vi "Dashboard Main.vi"() -> ()   [LabVIEW 2013]
uses:
  Program Files (x86)/National Instruments/LabVIEW 2013/examples/FRC/Vision/2014 Target Detection/TargetType.ctl
  <vilib>/event_ctls.llb/eventvkey.ctl
  <vilib>/Rock Robotics/WPI/Dashboard/WPI_DashboardLogging Global.vi
  <vilib>/Utility/config.llb/Write Key (String).vi
  <vilib>/Utility/config.llb/Write Key (I32).vi
  <vilib>/Utility/config.llb/NI_LVConfig.lvlib
panel:
  in  "Score Limit":dbl
  out "Target Info":T2(array[cluster])
  in  "Area Size Limit %":dbl=0.06 format="%#_13g"
  out "Image Message":string="Timeout in Camera Communications"
  in  "Rec Mode":enum32{"Stop", "Record", "Playback"}(radio)
  in  "Dashboard Tab":T3(tab)=enum."Auto"
  in  "Camera Settings":T4={"Frame Rate"=30, "Compression"=30, "Size"=1} {"Frame Rate" scale=1.0..30.0; "Size" items=["640x480", "320x240", "160x120"]}
  out "MotorSliders R":cluster{"MotorSlide1":dbl, "MotorSlide2":dbl} {"MotorSlide2" scale=-1.0..1.0 scale format="%#_2e"; "MotorSlide1" scale=-1.0..1.0 scale format="%#_2e"}
  out "MotorChart R":cluster{"Numeric":dbl, "Numeric":dbl}(graph)
  out "MotorSliders L":T5 {"MotorSlide4 2" scale=0.0..14.0 scale format="%#_2e"; "MotorSlide2" scale=-1.0..1.0 scale format="%#_2e"; "MotorSlide1" scale=-1.0..1.0 scale format="%#_2e"}
  out "MotorChart L":T6(graph)
  out "JS1 Z":dbl(slide) scale=-1.0..1.0 scale format="%#_2e"
  out "Joystick 1":cluster{"X":dbl, "Y":dbl}[](graph)
  out "JS Buttons 1":T7
  out "JS2 Z":dbl(slide) scale=-1.0..1.0 scale format="%#_2e"
  out "Joystick 2":cluster{"X":dbl, "Y":dbl}[](graph)
  out "JS Buttons 2":T7
  out "Mode":T8(ring)=enum."Auto Disabled"
  out "Camera IP":string
  in  "DB Camera Config":bool
  out "fps":dbl format="%#.1g"
  out "Mbps":dbl format="%#.1g"
  out "Mbps 2":bool
  out "LED 1":bool
  in  "Slider 1":dbl(slide) scale=0.0..100.0
  in  "Left?":bool
  in  "Checkbox 2":bool
  in  "Checkbox 1":bool
  in  "Color Components":T9={"Hue"={142.0, 183.0}, "Sat"={188.0, 255.0}, "Val"={0.0, 255.0}} {"Val" scale=0.0..255.0; "Sat" scale=0.0..255.0; "Hue" scale=0.0..255.0 scale format="%#_3g"}
  in  "Std Devs":cluster{"Hue":dbl, "Sat":dbl, "Val":dbl}={"Hue"=4.0, "Sat"=6.0, "Val"=4.0}
  in  "Score Cutoff":dbl(slide)=54.248366013071895 scale=0.0..100.0
  out "Distances":T10(array[cluster])
  out "State":T1
  in  "Test Slider":dbl(slide) scale=0.0..100.0 scale format="%#_3g"
  in  "On/Off":bool caption="Solenoid"
  in  "Test Name":u16(ring) items=["Select the test to run...", "Example Test", "-------------------------------", "List of tests is built in robot code.", "Replace with your own automated tests."]
  in  "Test Tree":string(tree)
  in  "Motor":cluster{"Value":dbl, "Enable":bool} {"Value" scale=-1.0..1.0 scale format="%#_3g"}
  out "Progress":T11 {"Test Progress" scale=0.0..100.0}
  in  "Rev/Fwd":cluster{"Forward":bool, "Reverse":bool}
  in  "Test Ring":u16(ring) items=["Auto", "Fixed indoor", "Fixed outdoor 1", "Fixed outdoor 2", "Fixed fluorescent 1", "Fixed fluorescent 2", "Hold current"]
  in  "Listbox":i32(listbox)
  out "Tree":string(tree)
  out "Camera Image":T12(plugin-control)
  in  "Enable":bool=TRUE
  # "Left"
  # "Front"
  # "Right"
  # "Battery"
  # "Customize by placing controls and indicators here and name to\nmatch Dashboard Variables on robot."
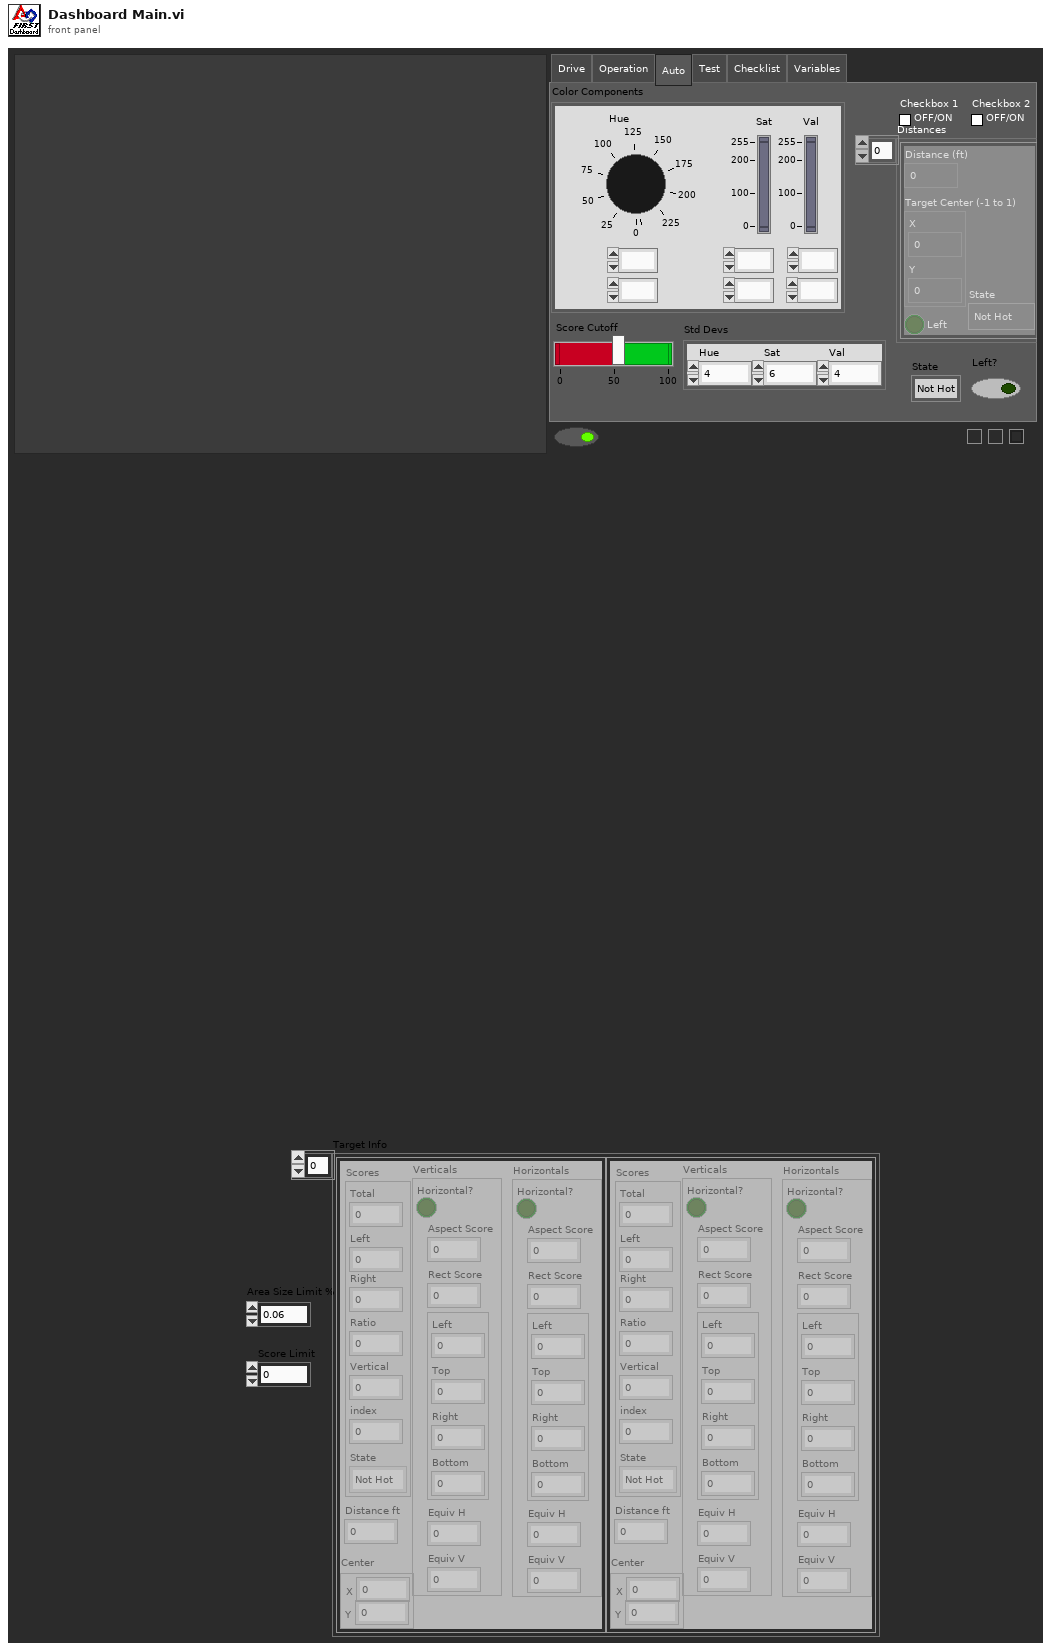
[diagram p1: front panel]
types:
  T1 = typedef "TargetType.ctl" = enum16{"Not Hot", "Hot"}
  T2 = cluster{"Scores":cluster{"Total":dbl, "Left":dbl, "Right":dbl, "Ratio":dbl, "Vertical":dbl, "index":i32, "State":T1}, "Verticals":cluster{"Horizontal?":bool, "Aspect Score":dbl, "Rect Score":dbl, cluster{"Left":dbl, "Top":dbl, "Right":dbl, "Bottom":dbl}, "Equiv H":dbl, "Equiv V":dbl}, "Horizontals":cluster{"Horizontal?":bool, "Aspect Score":dbl, "Rect Score":dbl, cluster{"Left":dbl, "Top":dbl, "Right":dbl, "Bottom":dbl}, "Equiv H":dbl, "Equiv V":dbl}, "Distance ft":dbl, "Center":cluster{"X":dbl, "Y":dbl}}[]
  T3 = enum32{"Drive", "Operation", "Auto", "Test", "Checklist", "Variables"}
  T4 = cluster{"Frame Rate":i32, "Compression":i32, "Size":u16}
  T5 = cluster{"MotorSlide1":dbl, "MotorSlide2":dbl, "MotorSlide4 2":dbl}
  T6 = cluster{"Numeric":dbl, "Numeric":dbl, "Battery":sgl}
  T7 = cluster{bool, bool, bool, bool, bool, bool, bool, bool, bool, bool, bool, bool}
  T8 = enum8{"Tele-Op Disabled", "Tele-Op Enabled", "Auto Disabled", "Auto Enabled", "Test Disabled", "Test Enabled", ""}
  T9 = cluster{"Hue":cluster{dbl, dbl}, "Sat":cluster{dbl, dbl}, "Val":cluster{dbl, dbl}}
  T10 = cluster{"Distance (ft)":dbl, "Target Center (-1 to 1)":cluster{"X":dbl, "Y":dbl}, "Left":bool, "State":T1}[]
  T11 = cluster{"Test Progress":u8, "Test Progress Text":string}
  T12 = typedef "IMAQ Image.ctl" = refnum<image>
  T13 = typedef "Image Type" = u32
  T14 = cluster{"Horizontal":bool, "Aspect Score":dbl, "Rect Score":dbl, cluster{"Left":dbl, "Top":dbl, "Right":dbl, "Bottom":dbl}, "Equiv H":dbl, "Equiv V":dbl}[]
  T15 = cluster{"Scores":cluster{"Total":dbl, "Left":dbl, "Right":dbl, "Ratio":dbl, "Vertical":dbl, "index":i32, "State":T1}, "Verticals":cluster{"Horizontal?":bool, "Aspect Score":dbl, "Rect Score":dbl, cluster{"Left":dbl, "Top":dbl, "Right":dbl, "Bottom":dbl}, "Equiv H":dbl, "Equiv V":dbl}, "Horizontals":cluster{"Horizontal?":bool, "Aspect Score":dbl, "Rect Score":dbl, cluster{"Left":dbl, "Top":dbl, "Right":dbl, "Bottom":dbl}, "Equiv H":dbl, "Equiv V":dbl}, "Validated":bool}[]
  T16 = cluster{"Scores":cluster{"Total":dbl, "Left":dbl, "Right":dbl, "Ratio":dbl, "Vertical":dbl, "index":i32, "State":T1}, "Verticals":cluster{"Horizontal?":bool, "Aspect Score":dbl, "Rect Score":dbl, cluster{"Left":dbl, "Top":dbl, "Right":dbl, "Bottom":dbl}, "Equiv H":dbl, "Equiv V":dbl}, "Horizontals":cluster{"Horizontal?":bool, "Aspect Score":dbl, "Rect Score":dbl, cluster{"Left":dbl, "Top":dbl, "Right":dbl, "Bottom":dbl}, "Equiv H":dbl, "Equiv V":dbl}, "Distance (ft)":dbl, "Target Center (-1 to 1)":cluster{"X":dbl, "Y":dbl}}[]
  T17 = cluster{"Target Info[0]":cluster{"Scores":cluster{"Total":dbl, "Left":dbl, "Right":dbl, "Ratio":dbl, "Vertical":dbl, "index":i32, "State":T1}, "Verticals":cluster{"Horizontal?":bool, "Aspect Score":dbl, "Rect Score":dbl, cluster{"Left":dbl, "Top":dbl, "Right":dbl, "Bottom":dbl}, "Equiv H":dbl, "Equiv V":dbl}, "Horizontals":cluster{"Horizontal?":bool, "Aspect Score":dbl, "Rect Score":dbl, cluster{"Left":dbl, "Top":dbl, "Right":dbl, "Bottom":dbl}, "Equiv H":dbl, "Equiv V":dbl}, "Distance (ft)":dbl, "Target Center (-1 to 1)":cluster{"X":dbl, "Y":dbl}}, "Target Info[1]":cluster{"Scores":cluster{"Total":dbl, "Left":dbl, "Right":dbl, "Ratio":dbl, "Vertical":dbl, "index":i32, "State":T1}, "Verticals":cluster{"Horizontal?":bool, "Aspect Score":dbl, "Rect Score":dbl, cluster{"Left":dbl, "Top":dbl, "Right":dbl, "Bottom":dbl}, "Equiv H":dbl, "Equiv V":dbl}, "Horizontals":cluster{"Horizontal?":bool, "Aspect Score":dbl, "Rect Score":dbl, cluster{"Left":dbl, "Top":dbl, "Right":dbl, "Bottom":dbl}, "Equiv H":dbl, "Equiv V":dbl}, "Distance (ft)":dbl, "Target Center (-1 to 1)":cluster{"X":dbl, "Y":dbl}}, "Target Info[2]":cluster{"Scores":cluster{"Total":dbl, "Left":dbl, "Right":dbl, "Ratio":dbl, "Vertical":dbl, "index":i32, "State":T1}, "Verticals":cluster{"Horizontal?":bool, "Aspect Score":dbl, "Rect Score":dbl, cluster{"Left":dbl, "Top":dbl, "Right":dbl, "Bottom":dbl}, "Equiv H":dbl, "Equiv V":dbl}, "Horizontals":cluster{"Horizontal?":bool, "Aspect Score":dbl, "Rect Score":dbl, cluster{"Left":dbl, "Top":dbl, "Right":dbl, "Bottom":dbl}, "Equiv H":dbl, "Equiv V":dbl}, "Distance (ft)":dbl, "Target Center (-1 to 1)":cluster{"X":dbl, "Y":dbl}}, "Target Info[3]":cluster{"Scores":cluster{"Total":dbl, "Left":dbl, "Right":dbl, "Ratio":dbl, "Vertical":dbl, "index":i32, "State":T1}, "Verticals":cluster{"Horizontal?":bool, "Aspect Score":dbl, "Rect Score":dbl, cluster{"Left":dbl, "Top":dbl, "Right":dbl, "Bottom":dbl}, "Equiv H":dbl, "Equiv V":dbl}, "Horizontals":cluster{"Horizontal?":bool, "Aspect Score":dbl, "Rect Score":dbl, cluster{"Left":dbl, "Top":dbl, "Right":dbl, "Bottom":dbl}, "Equiv H":dbl, "Equiv V":dbl}, "Distance (ft)":dbl, "Target Center (-1 to 1)":cluster{"X":dbl, "Y":dbl}}, "Target Info[4]":cluster{"Scores":cluster{"Total":dbl, "Left":dbl, "Right":dbl, "Ratio":dbl, "Vertical":dbl, "index":i32, "State":T1}, "Verticals":cluster{"Horizontal?":bool, "Aspect Score":dbl, "Rect Score":dbl, cluster{"Left":dbl, "Top":dbl, "Right":dbl, "Bottom":dbl}, "Equiv H":dbl, "Equiv V":dbl}, "Horizontals":cluster{"Horizontal?":bool, "Aspect Score":dbl, "Rect Score":dbl, cluster{"Left":dbl, "Top":dbl, "Right":dbl, "Bottom":dbl}, "Equiv H":dbl, "Equiv V":dbl}, "Distance (ft)":dbl, "Target Center (-1 to 1)":cluster{"X":dbl, "Y":dbl}}, "Target Info[5]":cluster{"Scores":cluster{"Total":dbl, "Left":dbl, "Right":dbl, "Ratio":dbl, "Vertical":dbl, "index":i32, "State":T1}, "Verticals":cluster{"Horizontal?":bool, "Aspect Score":dbl, "Rect Score":dbl, cluster{"Left":dbl, "Top":dbl, "Right":dbl, "Bottom":dbl}, "Equiv H":dbl, "Equiv V":dbl}, "Horizontals":cluster{"Horizontal?":bool, "Aspect Score":dbl, "Rect Score":dbl, cluster{"Left":dbl, "Top":dbl, "Right":dbl, "Bottom":dbl}, "Equiv H":dbl, "Equiv V":dbl}, "Distance (ft)":dbl, "Target Center (-1 to 1)":cluster{"X":dbl, "Y":dbl}}, "Target Info[6]":cluster{"Scores":cluster{"Total":dbl, "Left":dbl, "Right":dbl, "Ratio":dbl, "Vertical":dbl, "index":i32, "State":T1}, "Verticals":cluster{"Horizontal?":bool, "Aspect Score":dbl, "Rect Score":dbl, cluster{"Left":dbl, "Top":dbl, "Right":dbl, "Bottom":dbl}, "Equiv H":dbl, "Equiv V":dbl}, "Horizontals":cluster{"Horizontal?":bool, "Aspect Score":dbl, "Rect Score":dbl, cluster{"Left":dbl, "Top":dbl, "Right":dbl, "Bottom":dbl}, "Equiv H":dbl, "Equiv V":dbl}, "Distance (ft)":dbl, "Target Center (-1 to 1)":cluster{"X":dbl, "Y":dbl}}, "Target Info[7]":cluster{"Scores":cluster{"Total":dbl, "Left":dbl, "Right":dbl, "Ratio":dbl, "Vertical":dbl, "index":i32, "State":T1}, "Verticals":cluster{"Horizontal?":bool, "Aspect Score":dbl, "Rect Score":dbl, cluster{"Left":dbl, "Top":dbl, "Right":dbl, "Bottom":dbl}, "Equiv H":dbl, "Equiv V":dbl}, "Horizontals":cluster{"Horizontal?":bool, "Aspect Score":dbl, "Rect Score":dbl, cluster{"Left":dbl, "Top":dbl, "Right":dbl, "Bottom":dbl}, "Equiv H":dbl, "Equiv V":dbl}, "Distance (ft)":dbl, "Target Center (-1 to 1)":cluster{"X":dbl, "Y":dbl}}, "Target Info[8]":cluster{"Scores":cluster{"Total":dbl, "Left":dbl, "Right":dbl, "Ratio":dbl, "Vertical":dbl, "index":i32, "State":T1}, "Verticals":cluster{"Horizontal?":bool, "Aspect Score":dbl, "Rect Score":dbl, cluster{"Left":dbl, "Top":dbl, "Right":dbl, "Bottom":dbl}, "Equiv H":dbl, "Equiv V":dbl}, "Horizontals":cluster{"Horizontal?":bool, "Aspect Score":dbl, "Rect Score":dbl, cluster{"Left":dbl, "Top":dbl, "Right":dbl, "Bottom":dbl}, "Equiv H":dbl, "Equiv V":dbl}, "Distance (ft)":dbl, "Target Center (-1 to 1)":cluster{"X":dbl, "Y":dbl}}}
  T18 = cluster{cluster{dbl, dbl}, cluster{dbl, dbl}, cluster{dbl, dbl}}
  T19 = cluster{"Scores":cluster{"Total":dbl, "Left":dbl, "Right":dbl, "Ratio":dbl, "Vertical":dbl, "index":i32, "State":T1}, "Verticals":cluster{"Horizontal?":bool, "Aspect Score":dbl, "Rect Score":dbl, cluster{"Left":dbl, "Top":dbl, "Right":dbl, "Bottom":dbl}, "Equiv H":dbl, "Equiv V":dbl}, "Horizontals":cluster{"Horizontal?":bool, "Aspect Score":dbl, "Rect Score":dbl, cluster{"Left":dbl, "Top":dbl, "Right":dbl, "Bottom":dbl}, "Equiv H":dbl, "Equiv V":dbl}, "Distance (ft)":dbl, "Target Center (-1 to 1)":cluster{"X":dbl, "Y":dbl}}
  T20 = cluster{"Total":dbl, "Left":dbl, "Right":dbl, "Ratio":dbl, "Vertical":dbl, "index":i32, "State":T1}
  T21 = cluster{"Digital Inputs":bool[], "Digital Outputs":bool[]}
  T22 = cluster{"Competition mode":bool, "Robot Link":bool, "Autonomous":bool, "Enabled":bool, "E-Stop":bool, "Simulated":bool, "TestMode":bool, "Docked Window":bool}
  T23 = cluster{"Boolean Array[0]":bool, "Boolean Array[1]":bool, "Boolean Array[2]":bool, "Boolean Array[3]":bool, "Boolean Array[4]":bool, "Boolean Array[5]":bool, "Boolean Array[6]":bool, "Boolean Array[7]":bool, "Boolean Array[8]":bool, "Boolean Array[9]":bool, "Boolean Array[10]":bool, "Boolean Array[11]":bool}
  T24 = typedef "NI_LVConfig.lvlib/Config Data RefNum.ctl" = refnum<k1>
  T25 = typedef "eventvkey.ctl" = enum16{"ASCII", "Enter", "Return", "Shift", "Ctrl", "Alt", "Cmd", "Opt", "Caps", "NumLock", "Clear", "Break", "Up", "Down", "Left", "Right", "Insert", "Delete", "Home", "End", "PageUp", "PageDown", "Escape", "Help", "Pause", "ScrollLock", "F1", "F2", "F3", "F4", "F5", "F6", "F7", "F8", "F9", "F10", "F11", "F12", "F13", "F14", "F15", "F16", "F17", "F18", "F19", "F20", "F21", "F22", "F23", "F24", "Play", "VolumeUp", "VolumeDown", "Mute", "Two Byte Char"}
  T26 = cluster{"Image Size":bool, "Image Type":bool, "Pixel Value":bool, "ROI Information":bool, "Zoom Factor":bool}
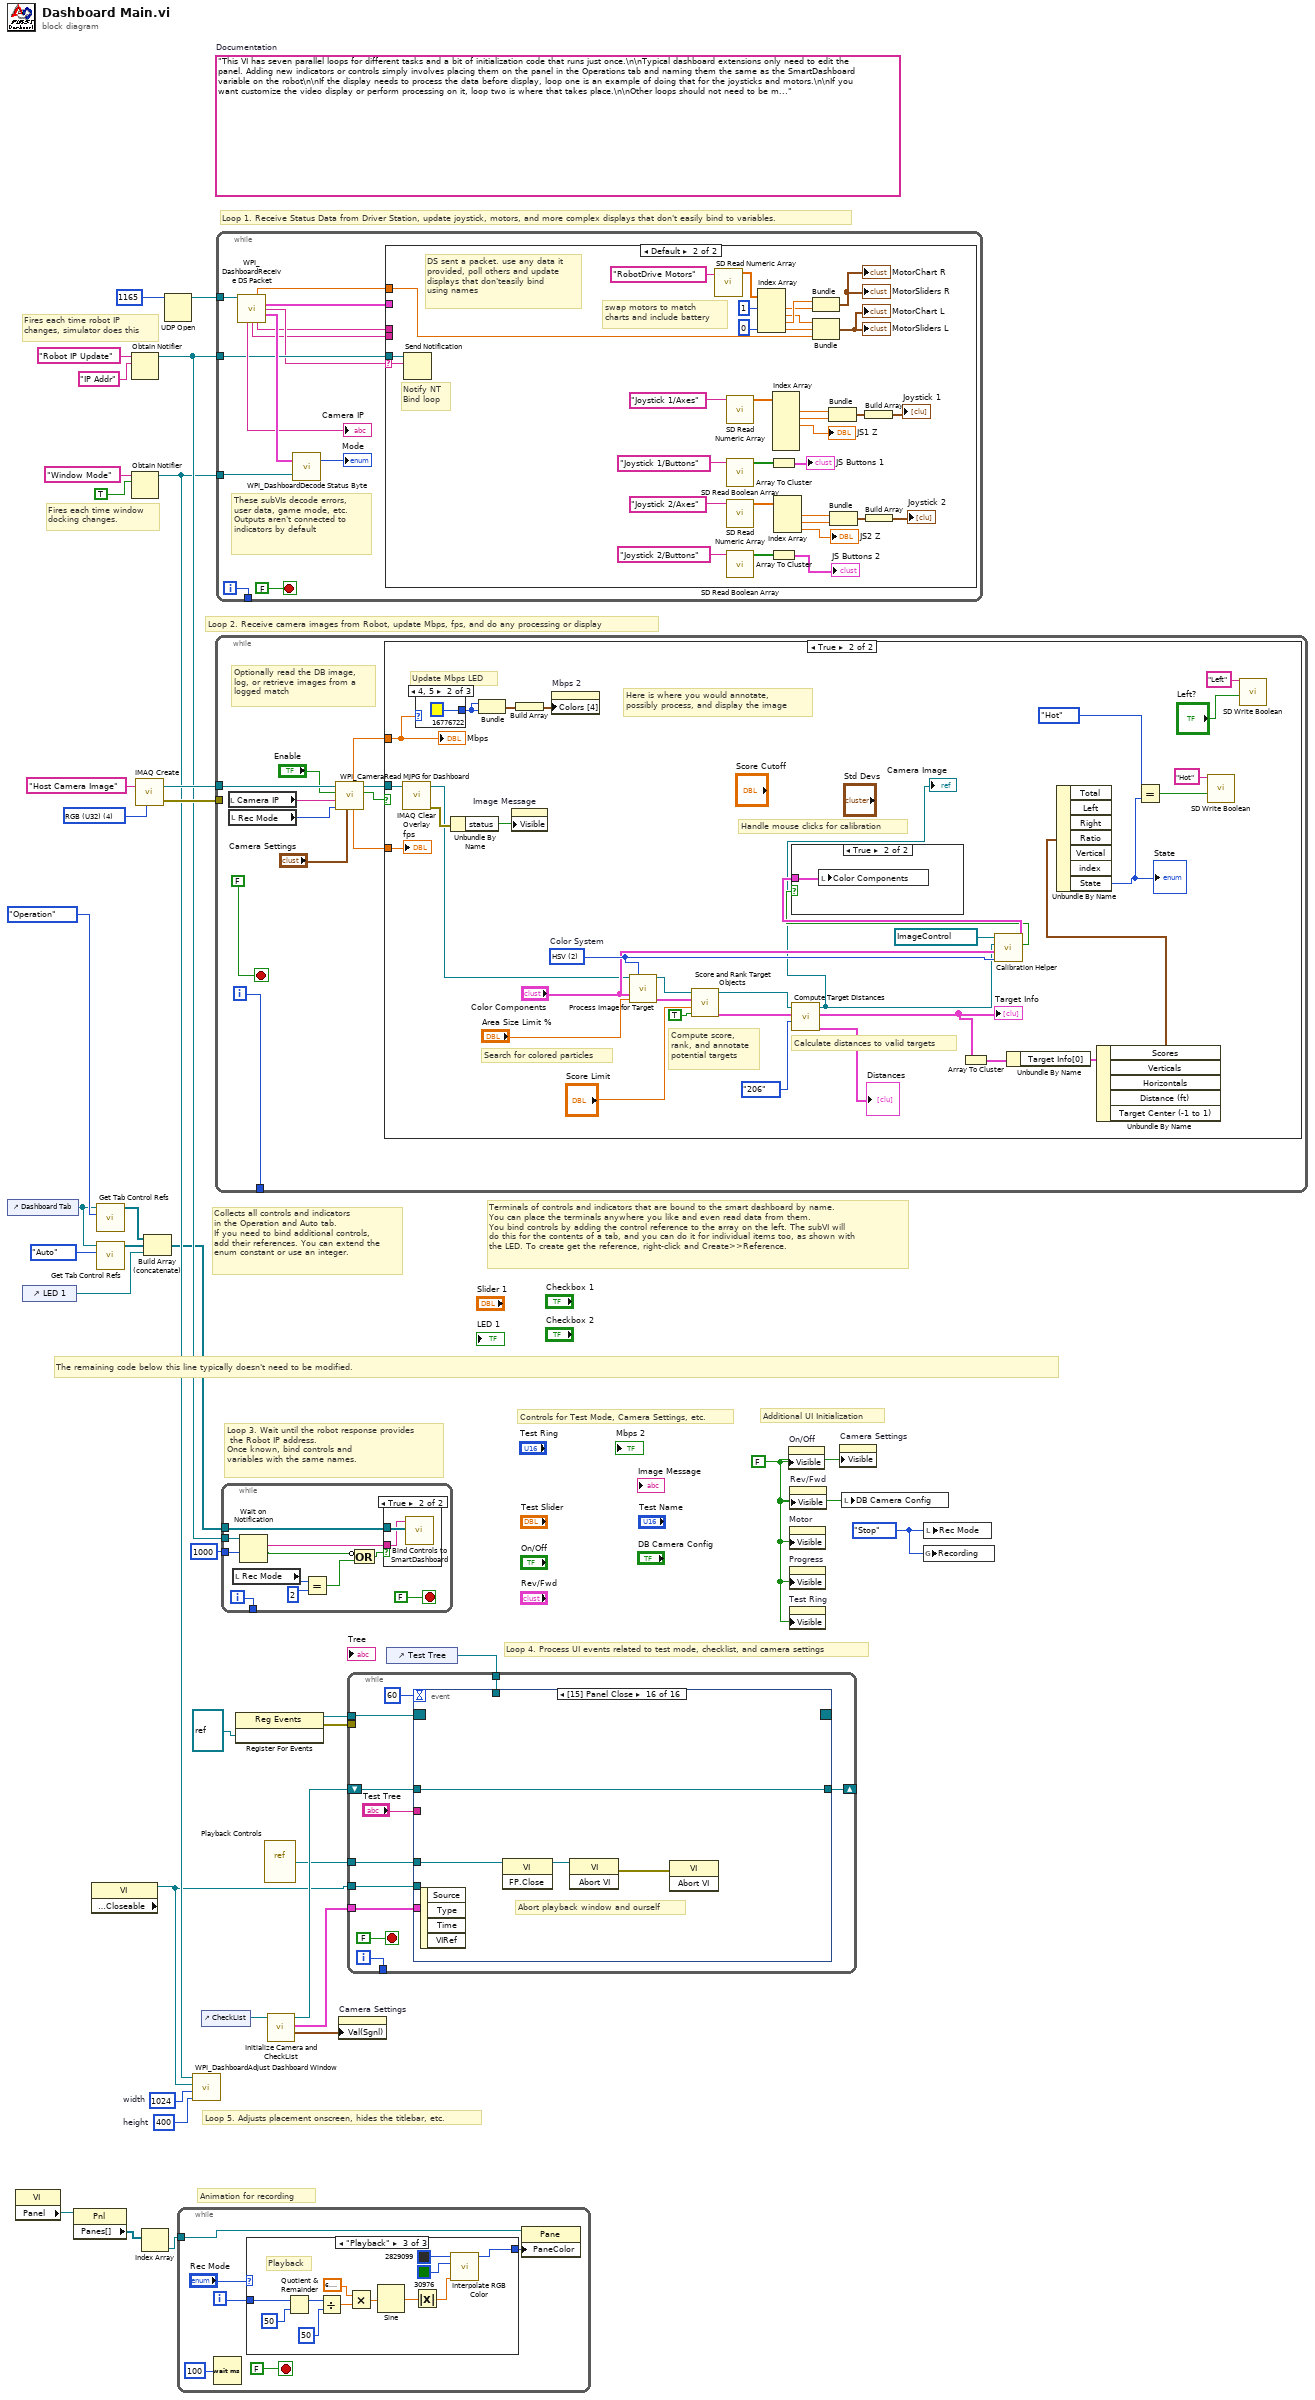
[diagram p0: block diagram]
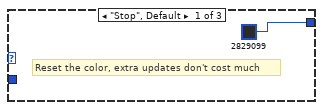
[diagram p2: hidden frame]
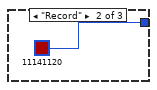
[diagram p3: hidden frame]
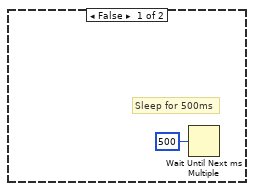
[diagram p5: hidden frame]
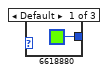
[diagram p7: hidden frame]
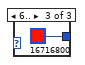
[diagram p8: hidden frame]
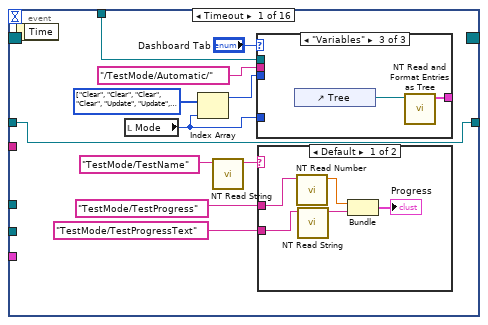
[diagram p9: hidden frame]
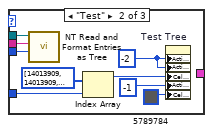
[diagram p11: hidden frame]
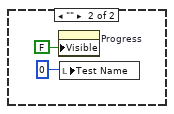
[diagram p12: hidden frame]
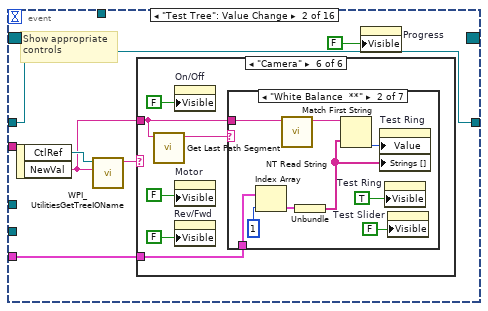
[diagram p13: hidden frame]
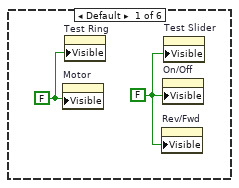
[diagram p14: hidden frame]
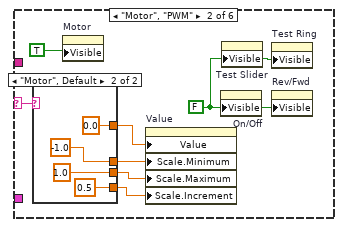
[diagram p15: hidden frame]
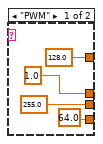
[diagram p16: hidden frame]
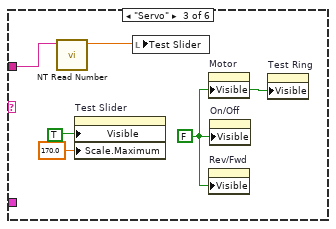
[diagram p17: hidden frame]
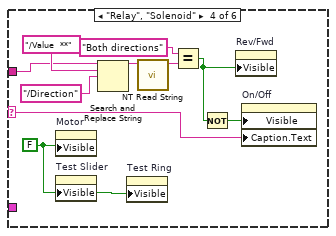
[diagram p18: hidden frame]
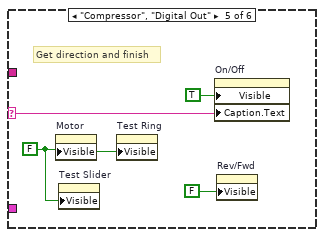
[diagram p19: hidden frame]
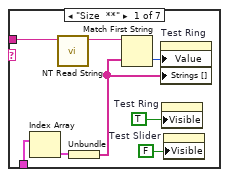
[diagram p20: hidden frame]
diagram:
  w8 = enum32{"Stop", "Record", "Playback"}."Stop" ("Rec Mode")
  w11 = 400  # height
  w12 = 1024  # width
  w25 = FALSE ("Visible")
  (unwired) "This VI has seven parallel loops for different tasks and a bit of initialization code that runs just once.\n\nTypical dashboard extensions only need to edit the panel. Adding new indicators or controls simply involves placing them on the panel in the Operations tab and naming them the same as the SmartDashboard variable on the robot\n\nIf the display needs to process the data before display, loop one is an example of doing that for the joysticks and motors.\n\nIf you want customize the video display or perform processing on it, loop two is where that takes place.\n\nOther loops should not need to be modified. They are pretty standard, and document the task they perform."  # Documentation
  w35 = T13 4 items=["Grayscale (U8)", "Grayscale (I16)", "Grayscale (SGL)", "Complex (CSG)", "RGB (U32)", "HSL (U32)", "RGB (U64)"] ("Image Type")
  # "Controls for Test Mode, Camera Settings, etc."
  # "Additional UI Initialization"
  # "Animation for recording"
  # "Fires each time robot IP\nchanges, simulator does this"
  # "Fires each time window\ndocking changes."
  # "Collects all controls and indicators\nin the Operation and Auto tab.\nIf you need to bind additional controls,\nadd their references. You can extend the\nenum constant or use an integer."
  # "The remaining code below this line typically doesn't need to be modified."
  # "Loop 4. Process UI events related to test mode, checklist, and camera settings"
  # "Terminals of controls and indicators that are bound to the smart dashboard by name.\nYou can place the terminals anywhere you like and even read data from them.\nYou bind controls by adding the control reference to the array on the left. The subVI will\ndo this for the contents of a tab, and you can do it for individual items too, as shown with\nthe LED. To create get the reference, right-click and Create>>Reference."
  # "Loop 3. Wait until the robot response provides\n the Robot IP address.\nOnce known, bind controls and\nvariables with the same names."
  # "Loop 5. Adjusts placement onscreen, hides the titlebar, etc."
  # "Loop 1. Receive Status Data from Driver Station, update joystick, motors, and more complex displays that don't easily bind to variables."
  # "Loop 2. Receive camera images from Robot, update Mbps, fps, and do any processing or display"
  n1 = control-ref of="Dashboard Tab"() -> (w6:refnum<vi>)
  n2 = property class="VI"() -> ("Panel"=w19:refnum<vi>)  [unwired: 2 in, 2 out]
  n3 = control-ref of="LED 1"() -> (w1:refnum<vi>)
  n4 = property class="Pnl"(reference=w19) -> ("Panes[]"=w20:refnum<vi>[])  [unwired: 1 in, 2 out]
  n5 = property class="VI" props=["Front Panel.Closeable"]() -> (reference out=w7:refnum<vi>)  [unwired: 2 in, 2 out]
  n6 = call <vilib>:"Get Tab Control Refs.vi"("Page Index"=T3."Operation" ("Dashboard Tab"), "TabControl in"=w6) -> ("ControlsOnPage"=w4:refnum<vi>[])  [unwired: 9 in]
  n7 = call <vilib>:"Get Tab Control Refs.vi"("Page Index"=T3."Auto" ("Dashboard Tab"), "TabControl in"=w6) -> ("ControlsOnPage"=w5:refnum<vi>[])  [unwired: 9 in]
  n8 = Obtain Notifier(name (unnamed)="Robot IP Update", notification data type="IP Addr" ("name (unnamed)")) -> (notifier out=w29:refnum<notifier>)  [unwired: 2 in, 2 out]
  n9 = Obtain Notifier(name (unnamed)="Window Mode", notification data type=TRUE) -> (notifier out=w10:refnum<notifier>)  [unwired: 2 in, 2 out]
  n10 = call "IMAQ Create"("Image Name"="Host Camera Image", "Image Type"=w35) -> ("New Image"=w33:T12, "error out"=w32:errorcluster)  [unwired: 2 in, 1 out]
  n11 = Index Array(array=w20) -> (element=w18:refnum<vi>)  [unwired: 1 in]
  n12 = Build Array (concatenate)(w4, w5, w1) -> (w3:refnum<vi>[])
  n13 = UDP Open(11:u16 1165 ("port")) -> (port=w36:refnum<k16>)  [unwired: 2 in, 4 out]
  n14 = while {
    tunnel: w18 -> [w39]
    i -> [w42]
    stop <- FALSE stop-if-true
    n15 = Wait (ms)(milliseconds to wait=u32 100) -> ()  [unwired: 1 out]
    n16 = case shown="\"Playback\"" "Rec Mode" {
      tunnel: w42 -> [_ _ w57]
      tunnel: [u32 2829099 ("Base Color") u32 11141120 ("Target Color") w46] -> w38
      frame "Stop", Default {
        # "Reset the color, extra updates don't cost much"
      }
      frame "Record" {
      }
      frame "Playback" {
        # "Playback"
        n17 = Quotient & Remainder(x=w57, y=u32 50 ("milliseconds to wait")) -> (x-y*floor(x/y)=w53:u32)  [unwired: 1 out]
        n18 = Divide(x=w53, y=u32 50 ("milliseconds to wait")) -> (x/y=w50:dbl)
        n19 = Multiply(x=6.283185307179586, y=w50) -> (x*y=w55:dbl)
        n20 = Sine(x=w55) -> (sin(x)=w54:dbl)
        n21 = Absolute Value(x=w54) -> (abs(x)=w47:dbl)
        n22 = call "Interpolate RGB Color.vi"("Proportion"=w47, "Target Color"=u32 30976, "Base Color"=u32 2829099) -> ("Result Color"=w46:u32)  [unwired: 8 in]
      }
    }
    n23 = property class="Pane"(reference=w39, "PaneColor"=w38) -> ()  [unwired: 1 in, 2 out]
  }
  n24 = call <vilib>:"WPI_DashboardAdjust Dashboard Window.vi"("height"=w11, "width"=w12, "reference in"=w7, "Notifier in"=w10) -> ()  [unwired: 8 in]
  n25 = control-ref of="CheckList"() -> (w9:refnum<vi>)
  n26 = while {
    tunnel: w33 -> [w66]
    tunnel: w32 -> [_]
    tunnel: [w67] -> _
    i -> [w67]
    stop <- FALSE stop-if-true
    # "Optionally read the DB image,\nlog, or retrieve images from a\nlogged match"
    n27 = local read "Camera IP"() -> (w59:string)
    n28 = local read "Rec Mode"() -> (w58:enum32{"Stop", "Record", "Playback"})
    n29 = call <vilib>:"WPI_CameraRead MJPG for Dashboard.vi"("Camera Settings"="Camera Settings", "Rec Mode"=w58, "Camera IP"=w59, "Enable"="Enable", "Refnum in"=w66) -> ("Active"=w63:bool, "Refnum out"=w65:T12, "FPS"=w62:dbl, "Bandwidth (Mbps)"=w61:dbl)  [unwired: 3 in]
    n30 = case shown="True" w63 {
      tunnel: w65 -> [_ w98]
      tunnel: w61 -> [_ w97]
      tunnel: w62 -> [_ w96]
      frame False {
        # "Sleep for 500ms"
        n31 = Wait Until Next ms Multiple(millisecond multiple=u32 500) -> ()  [unwired: 1 out]
      }
      frame True {
        w91 = u16 2 items=["RGB", "HSL", "HSV", "HSI"]  # Color System
        # "Calculate distances to valid targets"
        # "Search for colored particles"
        # "Handle mouse clicks for calibration"
        # "Compute score,\nrank, and annotate\npotential targets"
        # "Here is where you would annotate,\npossibly process, and display the image"
        # "Update Mbps LED"
        n32 = call "IMAQ Clear Overlay"("Image"=w98) -> ("error out"=w102:errorcluster, "Image Out"=w86:T12)  [unwired: 2 in, 7 out]
        n33 = case shown="4, 5" w97 {
          tunnel: [u32 6618880 ("Color Box") u32 16776722 ("Color Box") u32 16716800 ("Color Box")] -> w99
          frame Default {
          }
          frame 4, 5 {
          }
          frame 6.. {
          }
        }
        n34 = Unbundle By Name(w102) -> ("status"=w103:bool)
        n35 = Bundle("Color Box"=w99, "Color Box"=w99) -> (w101:cluster{"Color Box":u32, "Color Box":u32})  [unwired: 1 out]
        n36 = property on="Image Message" class="Str"("Visible"=w103) -> ()  [unwired: 2 in, 2 out]
        n37 = Build Array(w101) -> (w100:cluster{"Color Box":u32, "Color Box":u32}[])
        n38 = property on="Mbps 2" class="Bool (strict)"("Colors [4]"=w100) -> ()  [unwired: 2 in, 2 out]
        n39 = call "Process Image for Target.vi"("Src Image"=w86, "Color Mode"=w91, "Color Components"="Color Components", "Area Cutoff %"="Area Size Limit %") -> ("Src Image Out"=w94:T12, "Particles"=w93:T14)  [unwired: 9 in, 1 out]
        n40 = call "Score and Rank Target Objects.vi"("Annotate"=TRUE, "Score Limit"="Score Limit", "Particles"=w93, "Image in"=w94) -> ("Target Info"=w92:T15, "Annotated Image"=w85:T12)  [unwired: 6 in]
        n41 = call "Compute Target Distances.vi"("Camera Type"=enum16{"206", "1011", "1013"}."206", "Target Info"=w92, "Image in"=w85) -> ("Distances"=→"Distances":T10, "Target Info"=w79:T16, "Image out"=w84:T12)  [unwired: 6 in]
        "Camera Image" <- w84
        "Target Info" <- w79
        n42 = Array To Cluster(array=w79) -> (cluster=w80:T17)
        n43 = call "Calibration Helper.vi"("Color Mode"=w91, "Color Components"="Color Components", "Image"=w84, "Image Ctl Refnum"=refnum<vi> refnum) -> ("Changed"=w88:bool, "output color"=w90:T18)  [unwired: 6 in]
        n44 = case shown="True" w88 {
          tunnel: w90 -> [_ w104]
          frame False {
          }
          frame True {
            n45 = local write "Color Components"(w104) -> ()
          }
        }
        n46 = Unbundle By Name(w80) -> ("Target Info[0]"=w78:T19)
        n47 = Unbundle By Name(w78) -> ("Scores"=w77:T20)  [unwired: 4 out]
        n48 = Unbundle By Name(w77) -> ("State"=w75:T1)  [unwired: 6 out]
        "State" <- w75
        n49 = Equal?(x=TargetType."Hot" ("State"), y=w75) -> (x = y?=w73:bool)
        n50 = call <vilib>:"SD Write Boolean.vi"("Boolean"=w73, "Name"="Hot") -> ()  [unwired: 8 in, 2 out]
        n51 = call <vilib>:"SD Write Boolean.vi"("Boolean"="Left?", "Name"="Left") -> ()  [unwired: 8 in, 2 out]
        "Mbps" <- w97
        "fps" <- w96
      }
    }
  }
  n52 = while {
    tunnel: w36 -> [w118]
    tunnel: w29 -> [w113]
    tunnel: w10 -> [w117]
    tunnel: [w114] -> _
    i -> [w114]
    stop <- FALSE stop-if-true
    # "These subVIs decode errors, user data, game mode, etc.\nOutputs aren't connected to indicators by default"
    n53 = call <vilib>:"WPI_DashboardReceive DS Packet.vi"("Recv Socket"=w118) -> ("Battery"=w108:sgl, "Driver Station"=w109:T21, "Robot IP Address"=w112:string, "Status"=w119:T22, "Camera IP Address"=→"Camera IP":string, "Low Priority User Data"=w111:string, "High Priority User Data"=w110:string)  [unwired: 1 in, 7 out]
    n54 = call <vilib>:"WPI_DashboardDecode Status Byte.vi"("Window Mode Notifier"=w117, "Status"=w119) -> ("Mode"=→"Mode":T8)  [unwired: 1 out]
    n55 = case shown="Default" w112 {
      selector: w112 -> [_ w131]
      tunnel: w113 -> [_ w132]
      tunnel: w111 -> [_ _]
      tunnel: w110 -> [_ _]
      tunnel: w109 -> [_ _]
      tunnel: w108 -> [_ w130]
      frame "0.0.0.0" {
        # "DS not sending packets, or no robot exists yet.\nDon't poll the variables"
      }
      frame Default {
        # "Notify NT\nBind loop"
        # "DS sent a packet. use any data it\nprovided, poll others and update\ndisplays that don'teasily bind\nusing names"
        # "swap motors to match\ncharts and include battery"
        n56 = Send Notification(notification=w131, notifier=w132) -> ()  [unwired: 1 in, 2 out]
        n57 = call <vilib>:"SD Read Numeric Array.vi"("Name"="RobotDrive Motors") -> ("Numeric Array"=w129:dbl[])  [unwired: 8 in, 2 out]
        n58 = call <vilib>:"SD Read Numeric Array.vi"("Name"="Joystick 1/Axes") -> ("Numeric Array"=w148:dbl[])  [unwired: 8 in, 2 out]
        n59 = call <vilib>:"SD Read Boolean Array.vi"("Name"="Joystick 1/Buttons") -> ("Boolean Array"=w150:bool[])  [unwired: 8 in, 2 out]
        n60 = call <vilib>:"SD Read Numeric Array.vi"("Name"="Joystick 2/Axes") -> ("Numeric Array"=w142:dbl[])  [unwired: 8 in, 2 out]
        n61 = call <vilib>:"SD Read Boolean Array.vi"("Name"="Joystick 2/Buttons") -> ("Boolean Array"=w141:bool[])  [unwired: 8 in, 2 out]
        n62 = Index Array(array=w129, index #1=1, index #4=0) -> (element #1=w125:dbl, element #2=w124:dbl, element #3=w126:dbl, element #4=w121:dbl)  [unwired: 2 in]
        n63 = Array To Cluster(array=w150) -> (cluster=→"JS Buttons 1":T23)
        n64 = Array To Cluster(array=w141) -> (cluster=→"JS Buttons 2":T23)
        n65 = Index Array(array=w148) -> (element #1=w145:dbl, element #2=w146:dbl, element #3=→"JS1 Z":dbl)  [unwired: 6 in, 3 out]
        n66 = Index Array(array=w142) -> (element #1=w137:dbl, element #2=w136:dbl, element #3=→"JS2 Z":dbl)  [unwired: 3 in]
        n67 = Bundle("Numeric"=w126, "Numeric"=w125) -> (→"MotorChart R" →"MotorSliders R":cluster{"Numeric":dbl, "Numeric":dbl})  [unwired: 1 in]
        n68 = Bundle("Numeric"=w124, "Numeric"=w121, "Battery"=w130) -> (→"MotorChart L" →"MotorSliders L":T6)  [unwired: 1 in]
        n69 = Bundle("Numeric"=w145, "Numeric"=w146) -> (w144:cluster{"Numeric":dbl, "Numeric":dbl})  [unwired: 1 in]
        n70 = Bundle("Numeric"=w137, "Numeric"=w136) -> (w138:cluster{"Numeric":dbl, "Numeric":dbl})  [unwired: 1 in]
        n71 = Build Array(w144) -> (→"Joystick 1":cluster{"Numeric":dbl, "Numeric":dbl}[])
        n72 = Build Array(w138) -> (→"Joystick 2":cluster{"Numeric":dbl, "Numeric":dbl}[])
      }
    }
  }
  n73 = while {
    tunnel: w3 -> [w164]
    tunnel: w29 -> [w162]
    tunnel: [w160] -> _
    tunnel: u32 1000 ("milliseconds to wait") -> [w159]
    i -> [w160]
    stop <- FALSE stop-if-true
    n74 = local read "Rec Mode"() -> (w155:enum32{"Stop", "Record", "Playback"})
    n75 = Wait on Notification(notifier=w162, timeout in ms (-1)=w159) -> (notification=w161:string, timed out?=w157:bool)  [unwired: 2 in, 2 out]
    n76 = Equal?(x=w155, y=u16 2 ("Rec Mode")) -> (x = y?=w156:bool)
    n77 = Compound Arithmetic op=OR(invert w157, w156) -> (w158:bool)
    n78 = case shown="True" w158 {
      tunnel: w164 -> [_ w166]
      tunnel: w161 -> [_ w165]
      frame False {
      }
      frame True {
        n79 = call <vilib>:"Bind Controls to SmartDashboard.vi"("Bound Control Refs"=w166, "Server IP Address"=w165) -> ()  [unwired: 10 in]
      }
    }
  }
  n80 = register-events(refnum<vi> refnum) -> (reference out=w16:refnum<event-registration>, error out=w15:errorcluster)  [unwired: 2 in]
  n81 = vi-ref "Playback Controls.vi"() -> (w17:refnum<vi>)
  n82 = call "Initialize Camera and CheckList.vi"("ListBox in"=w9) -> ("Cluster"=w23:cluster{"value":i32, "value":i32, "index":i32}, "Array"=w24:cluster{string[]}[], "File Refnum"=w22:T24)  [unwired: 8 in]
  n83 = property on="Camera Settings" class="Clust (strict)"("Val(Sgnl)"=w23) -> ()  [unwired: 2 in, 2 out]
  n84 = control-ref of="Test Tree"() -> (w21:refnum<vi>)
  n85 = while {
    tunnel: w24 -> [w174]
    shift-right: [w173] -> _
    shift-left: w22 -> [w172]
    tunnel: [w171] -> _
    tunnel: w21 -> [w170]
    tunnel: w17 -> [w169]
    tunnel: w16 -> [w168]
    tunnel: w15 -> [_]
    tunnel: w7 -> [w167]
    i -> [w171]
    stop <- FALSE stop-if-true
    n86 = event shown="[15] Panel Close" {
      selector: w168 -> [_ _ _ _ _ _ _ _ _ _ _ _ _ _ _ _]
      dyn-events: [_ _ _ _ _ _ _ _ _ _ _ _ _ w412 _ _] -> _
      timeout: u32 60 ("milliseconds to wait") -> [_ _ _ _ _ _ _ _ _ _ _ _ _ _ _ _]
      tunnel: w170 -> [w184 _ _ _ _ _ _ _ _ _ _ _ _ _ _ _]
      tunnel: "Test Tree" -> [_ _ _ _ _ _ _ _ w381 w389 w391 w395 w403 _ _ _]
      tunnel: w174 -> [_ w208 _ _ _ _ w345 w375 _ _ _ _ _ _ _ _]
      tunnel: [w178 w207 w306 w311 w319 w331 w344 w368 w380 w387 w390 w394 w402 w414 w428 w429] -> w173
      tunnel: w172 -> [w178 w207 w306 w311 w319 w331 w343 w368 w380 w387 w390 w394 w402 w414 w428 w429]
      tunnel: w169 -> [_ _ _ _ _ _ _ _ _ _ _ _ _ w415 _ w432]
      tunnel: w167 -> [_ _ _ _ _ _ _ _ _ _ _ _ _ w410 _ _]
      event Timeout {
        w183 = enum16{"Update", "Clear"}[] [enum."Clear", enum."Clear", enum."Clear", enum."Clear", enum."Update", enum."Update", enum."Clear"] items=["Update", "Clear"]
        n87 = event-data() -> ()  [unwired: 1 in, 1 out]
        n88 = local read "Mode"() -> (w181:T8)
        n89 = Index Array(array=w183, index=w181) -> (element=w182:enum16{"Update", "Clear"})
        n90 = call <vilib>:"NT Read String.vi"("Name"="TestMode/TestName") -> ("String"=w187:string)  [unwired: 9 in, 1 out]
        n91 = case shown="\"Variables\"" "Dashboard Tab" {
          tunnel: w184 -> [_ w197 _]
          tunnel: "/TestMode/Automatic/" ("Name Pattern") -> [_ w196 _]
          tunnel: w182 -> [_ w195 _]
          tunnel: w181 -> [_ w193 _]
          tunnel: [_ _ w199] -> _
          frame "Operation", Default {
          }
          frame "Test" {
            w192 = -2 ("Active Item:Row Number")
            n92 = call <vilib>:"NT Read and Format Entries as Tree.vi"("Operation"=w195, "Name Pattern"=w196, "Tree Refnum"=w197) -> ()  [unwired: 7 in, 2 out]
            n93 = Index Array(array=u32[] [14013909, 14013909, 14013909, 14013909, 14013909, 16777215, 14013909], index=w193) -> (element=w191:u32)
            n94 = property on="Test Tree" class="Tree (strict)"("Active Item Row Number"=w192, "ActiveColNum"=w192, "CellBG"=w191, "Active Item Row Number"=-1 ("Active Item:Row Number"), "CellBG"=u32 5789784 ("Color Box")) -> ()  [unwired: 2 in, 2 out]
          }
          frame "Variables" {
            n95 = control-ref of="Tree"() -> (w198:refnum<vi>)
            n96 = call <vilib>:"NT Read and Format Entries as Tree.vi"("Tree Refnum"=w198) -> ("Formatted Strings"=w199:cluster{"Name":string, "Value":string}[])  [unwired: 9 in, 1 out]
          }
        }
        n97 = case shown="Default" w187 {
          tunnel: "TestMode/TestProgress" ("Name") -> [w201 _]
          tunnel: "TestMode/TestProgressText" ("Name") -> [w200 _]
          frame Default {
            n98 = call <vilib>:"NT Read Number.vi"("Name"=w201) -> ("Numeric"=w202:dbl)  [unwired: 9 in, 1 out]
            n99 = call <vilib>:"NT Read String.vi"("Name"=w200) -> ("String"=w203:string)  [unwired: 9 in, 1 out]
            n100 = Bundle("Numeric"=w202, "String"=w203) -> (→"Progress":cluster{"Numeric":dbl, "String":string})  [unwired: 1 in]
          }
          frame "" {
            n101 = property on="Progress" class="Clust (strict)"("Visible"=FALSE) -> ()  [unwired: 2 in, 2 out]
            n102 = local write "Test Name"(u16 0) -> ()
          }
        }
      }
      event "Test Tree": Value Change {
        # "Show appropriate\ncontrols"
        n103 = event-data() -> ("CtlRef"=w211:refnum<vi>, "NewVal"=w209:string)  [unwired: 1 in]
        n104 = call <vilib>:"WPI_UtilitiesGetTreeIOName.vi"("NewVal"=w209, "TreeControl in"=w211) -> ("I/O Name"=w212:string)  [unwired: 9 in]
        n105 = case shown="\"Camera\"" w212 {
          selector: w212 -> [_ w219 _ w237 w246 _]
          tunnel: w209 -> [_ _ w234 w236 _ w253]
          tunnel: w208 -> [_ _ _ _ _ w252]
          frame Default {
            w214 = FALSE ("Visible")
            w213 = FALSE ("Visible")
            n106 = property on="Motor" class="Clust (strict)"("Visible"=w213) -> ()  [unwired: 2 in, 2 out]
            n107 = property on="Test Ring" class="Ring (strict)"("Visible"=w213) -> ()  [unwired: 2 in, 2 out]
            n108 = property on="Rev/Fwd" class="Clust (strict)"("Visible"=w214) -> ()  [unwired: 2 in, 2 out]
            n109 = property on="On/Off" class="Bool (strict)"("Visible"=w214) -> ()  [unwired: 2 in, 2 out]
            n110 = property on="Test Slider" class="Slide (strict)"("Visible"=w214) -> ()  [unwired: 2 in, 2 out]
          }
          frame "Motor", "PWM" {
            w220 = FALSE ("Visible")
            n111 = case shown="\"Motor\", Default" w219 {
              tunnel: [1.0 ("Value") -1.0 ("Value")] -> w218
              tunnel: [255.0 ("Value") 1.0 ("Value")] -> w217
              tunnel: [128.0 ("Value") 0.0 ("Value")] -> w216
              tunnel: [64.0 ("Value") 0.5 ("Value")] -> w215
              frame "PWM" {
              }
              frame "Motor", Default {
              }
            }
            n112 = property on="Motor" class="Clust (strict)"("Visible"=TRUE) -> ()  [unwired: 2 in, 2 out]
            n113 = property on="Value" class="Slide (strict)"("Value"=w216, "Scale.Minimum"=w218, "Scale.Maximum"=w217, "Scale.Increment"=w215) -> ()  [unwired: 2 in, 2 out]
            n114 = property on="On/Off" class="Bool (strict)"("Visible"=w220) -> ()  [unwired: 2 in, 2 out]
            n115 = property on="Test Slider" class="Slide (strict)"("Visible"=w220) -> ()  [unwired: 2 in, 2 out]
            n116 = property on="Test Ring" class="Ring (strict)"("Visible"=w220) -> ()  [unwired: 2 in, 2 out]
            n117 = property on="Rev/Fwd" class="Clust (strict)"("Visible"=w220) -> ()  [unwired: 2 in, 2 out]
          }
          frame "Servo" {
            w232 = FALSE ("Visible")
            n118 = call <vilib>:"NT Read Number.vi"("Name"=w234) -> ("Numeric"=w233:dbl)  [unwired: 9 in, 1 out]
            n119 = property on="Test Slider" class="Slide (strict)"("Visible"=TRUE, "Scale.Maximum"=170.0 ("Scale.Range:Maximum")) -> ()  [unwired: 2 in, 2 out]
            n120 = local write "Test Slider"(w233) -> ()
            n121 = property on="Motor" class="Clust (strict)"("Visible"=w232) -> ()  [unwired: 2 in, 2 out]
            n122 = property on="Rev/Fwd" class="Clust (strict)"("Visible"=w232) -> ()  [unwired: 2 in, 2 out]
            n123 = property on="On/Off" class="Bool (strict)"("Visible"=w232) -> ()  [unwired: 2 in, 2 out]
            n124 = property on="Test Ring" class="Ring (strict)"("Visible"=w232) -> ()  [unwired: 2 in, 2 out]
          }
          frame "Relay", "Solenoid" {
            w235 = FALSE ("Visible")
            n125 = property on="Motor" class="Clust (strict)"("Visible"=w235) -> ()  [unwired: 2 in, 2 out]
            n126 = property on="Test Slider" class="Slide (strict)"("Visible"=w235) -> ()  [unwired: 2 in, 2 out]
            n127 = Search and Replace String(input string=w236, search string="/Value  **", replace string="/Direction") -> (result string=w242:string)  [unwired: 5 in, 3 out]
            n128 = property on="Test Ring" class="Ring (strict)"("Visible"=w235) -> ()  [unwired: 2 in, 2 out]
            n129 = call <vilib>:"NT Read String.vi"("Name"=w242) -> ("String"=w240:string)  [unwired: 9 in, 1 out]
            n130 = Equal?(x="Both directions", y=w240) -> (x = y?=w238:bool)
            n131 = Not(x=w238) -> (.not. x?=w239:bool)
            n132 = property on="Rev/Fwd" class="Clust (strict)"("Visible"=w238) -> ()  [unwired: 2 in, 2 out]
            n133 = property on="On/Off" class="Bool (strict)"("Visible"=w239, "Caption.Text"=w237) -> ()  [unwired: 2 in, 2 out]
          }
          frame "Compressor", "Digital Out" {
            w245 = FALSE ("Visible")
            # "Get direction and finish"
            n134 = property on="Motor" class="Clust (strict)"("Visible"=w245) -> ()  [unwired: 2 in, 2 out]
            n135 = property on="Test Slider" class="Slide (strict)"("Visible"=w245) -> ()  [unwired: 2 in, 2 out]
            n136 = property on="Test Ring" class="Ring (strict)"("Visible"=w245) -> ()  [unwired: 2 in, 2 out]
            n137 = property on="On/Off" class="Bool (strict)"("Visible"=TRUE, "Caption.Text"=w246) -> ()  [unwired: 2 in, 2 out]
            n138 = property on="Rev/Fwd" class="Clust (strict)"("Visible"=FALSE) -> ()  [unwired: 2 in, 2 out]
          }
          frame "Camera" {
            n139 = call <vilib>:"Get Last Path Segment.vi"("String in"=w253) -> ("String out"=w254:string)  [unwired: 10 in]
            n140 = property on="On/Off" class="Bool (strict)"("Visible"=FALSE) -> ()  [unwired: 2 in, 2 out]
            n141 = property on="Motor" class="Clust (strict)"("Visible"=FALSE) -> ()  [unwired: 2 in, 2 out]
            n142 = property on="Rev/Fwd" class="Clust (strict)"("Visible"=FALSE) -> ()  [unwired: 2 in, 2 out]
            n143 = case shown="\"White Balance  **\"" w254 {
              tunnel: w253 -> [w260 w269 w278 w287 w296 _ w302]
              tunnel: w252 -> [w258 w266 w275 w284 w293 _ _]
              frame "Size  **" {
                n144 = Index Array(array=w258) -> (element=w257:cluster{string[]})  [unwired: 1 in]
                n145 = call <vilib>:"NT Read String.vi"("Name"=w260) -> ("String"=w259:string)  [unwired: 9 in, 1 out]
                n146 = Unbundle(w257) -> (w255:string[])
                n147 = Match First String(2:w255, 3:w259) -> (0:w256:i32)  [unwired: 1 out]
                n148 = property on="Test Ring" class="Ring (strict)"("Value"=w256, "Strings []"=w255) -> ()  [unwired: 2 in, 2 out]
                n149 = property on="Test Ring" class="Ring (strict)"("Visible"=TRUE) -> ()  [unwired: 2 in, 2 out]
                n150 = property on="Test Slider" class="Slide (strict)"("Visible"=FALSE) -> ()  [unwired: 2 in, 2 out]
              }
              frame "White Balance  **" {
                n151 = Index Array(array=w266, index=1) -> (element=w267:cluster{string[]})
                n152 = call <vilib>:"NT Read String.vi"("Name"=w269) -> ("String"=w268:string)  [unwired: 9 in, 1 out]
                n153 = Unbundle(w267) -> (w264:string[])
                n154 = Match First String(2:w264, 3:w268) -> (0:w263:i32)  [unwired: 1 out]
                n155 = property on="Test Ring" class="Ring (strict)"("Value"=w263, "Strings []"=w264) -> ()  [unwired: 2 in, 2 out]
                n156 = property on="Test Ring" class="Ring (strict)"("Visible"=TRUE) -> ()  [unwired: 2 in, 2 out]
                n157 = property on="Test Slider" class="Slide (strict)"("Visible"=FALSE) -> ()  [unwired: 2 in, 2 out]
              }
              frame "Exposure  **" {
                n158 = Index Array(array=w275, index=2) -> (element=w276:cluster{string[]})
                n159 = call <vilib>:"NT Read String.vi"("Name"=w278) -> ("String"=w277:string)  [unwired: 9 in, 1 out]
                n160 = Unbundle(w276) -> (w272:string[])
                n161 = Match First String(2:w272, 3:w277) -> (0:w273:i32)  [unwired: 1 out]
                n162 = property on="Test Ring" class="Ring (strict)"("Value"=w273, "Strings []"=w272) -> ()  [unwired: 2 in, 2 out]
                n163 = property on="Test Ring" class="Ring (strict)"("Visible"=TRUE) -> ()  [unwired: 2 in, 2 out]
                n164 = property on="Test Slider" class="Slide (strict)"("Visible"=FALSE) -> ()  [unwired: 2 in, 2 out]
              }
              frame "Exposure Priority  **" {
                n165 = Index Array(array=w284, index=3) -> (element=w285:cluster{string[]})
                n166 = call <vilib>:"NT Read String.vi"("Name"=w287) -> ("String"=w286:string)  [unwired: 9 in, 1 out]
                n167 = Unbundle(w285) -> (w281:string[])
                n168 = Match First String(2:w281, 3:w286) -> (0:w282:i32)  [unwired: 1 out]
                n169 = property on="Test Ring" class="Ring (strict)"("Value"=w282, "Strings []"=w281) -> ()  [unwired: 2 in, 2 out]
                n170 = property on="Test Ring" class="Ring (strict)"("Visible"=TRUE) -> ()  [unwired: 2 in, 2 out]
                n171 = property on="Test Slider" class="Slide (strict)"("Visible"=FALSE) -> ()  [unwired: 2 in, 2 out]
              }
              frame "Color Enable  **" {
                n172 = Index Array(array=w293, index=4) -> (element=w294:cluster{string[]})
                n173 = call <vilib>:"NT Read String.vi"("Name"=w296) -> ("String"=w295:string)  [unwired: 9 in, 1 out]
                n174 = Unbundle(w294) -> (w290:string[])
                n175 = Match First String(2:w290, 3:w295) -> (0:w291:i32)  [unwired: 1 out]
                n176 = property on="Test Ring" class="Ring (strict)"("Value"=w291, "Strings []"=w290) -> ()  [unwired: 2 in, 2 out]
                n177 = property on="Test Ring" class="Ring (strict)"("Visible"=TRUE) -> ()  [unwired: 2 in, 2 out]
                n178 = property on="Test Slider" class="Slide (strict)"("Visible"=FALSE) -> ()  [unwired: 2 in, 2 out]
              }
              frame Default {
                n179 = property on="Test Ring" class="Ring (strict)"("Visible"=FALSE) -> ()  [unwired: 2 in, 2 out]
                n180 = property on="Test Slider" class="Slide (strict)"("Visible"=FALSE) -> ()  [unwired: 2 in, 2 out]
              }
              frame "Brightness  **", "Color Level  **", "Compression  **", "FPS  **", "Sharpness  **" {
                n181 = call <vilib>:"NT Read Number.vi"("Name"=w302) -> ("Numeric"=w301:dbl)  [unwired: 9 in, 1 out]
                n182 = local write "Test Slider"(w301) -> ()
                n183 = property on="Test Slider" class="Slide (strict)"("Visible"=TRUE, "Scale.Maximum"=100.0 ("Scale.Range:Maximum")) -> ()  [unwired: 2 in, 2 out]
                n184 = property on="Test Ring" class="Ring (strict)"("Visible"=FALSE) -> ()  [unwired: 2 in, 2 out]
              }
            }
          }
        }
        n185 = property on="Progress" class="Clust (strict)"("Visible"=FALSE) -> ()  [unwired: 2 in, 2 out]
      }
      event "Test Name": Mouse Enter {
        # "Populate the ring with the list of tests"
        n186 = event-data() -> ()  [unwired: 1 in, 1 out]
        n187 = call <vilib>:"NT Read String Array.vi"("Name"="TestMode/TestList") -> ("String Array"=w310:string[])  [unwired: 9 in, 1 out]
        n188 = Build Array (concatenate)("Select the test to run...", w310) -> (w309:string[])
        n189 = property on="Test Name" class="Ring (strict)"("Strings []"=w309) -> ()  [unwired: 2 in, 2 out]
      }
      event "Test Name": Value Change {
        w312 = FALSE ("Visible")
        # "Tell the robot the test name to run"
        n190 = event-data() -> ("NewVal"=w316:u16)  [unwired: 1 in]
        n191 = property on="Test Name" class="Ring (strict)"() -> ("Strings []"=w317:string[])  [unwired: 2 in, 2 out]
        n192 = local write "Progress"(T11 {"Test Progress"=0, "Test Progress Text"=""} ("Progress")) -> ()
        n193 = Index Array(array=w317, index=w316) -> (element=w315:string)
        n194 = call <vilib>:"NT Write String.vi"("String"=w315, "Name"="TestMode/TestName") -> ()  [unwired: 9 in, 1 out]
        n195 = property on="Progress" class="Clust (strict)"("Visible"=TRUE) -> ()  [unwired: 2 in, 2 out]
        n196 = property on="Motor" class="Clust (strict)"("Visible"=w312) -> ()  [unwired: 2 in, 2 out]
        n197 = property on="Test Slider" class="Slide (strict)"("Visible"=w312) -> ()  [unwired: 2 in, 2 out]
        n198 = property on="On/Off" class="Bool (strict)"("Visible"=w312) -> ()  [unwired: 2 in, 2 out]
        n199 = property on="Rev/Fwd" class="Clust (strict)"("Visible"=w312) -> ()  [unwired: 2 in, 2 out]
        n200 = property on="Test Ring" class="Ring (strict)"("Visible"=w312) -> ()  [unwired: 2 in, 2 out]
      }
      event "Listbox": Double Click {
        n201 = event-data() -> ("PlatMods.Shift"=w320:bool, "Row"=w322:i32)  [unwired: 1 in]
        n202 = case shown="True" w320 {
          tunnel: w322 -> [w326 _]
          tunnel: 1 -> [w325 _]
          frame False {
            n203 = property on="Listbox" class="LstBox (strict)"() -> ("Item Symbols"=w324:i32[])  [unwired: 2 in, 2 out]
            n204 = Replace Array Subset(array=w324, new element=w325, index=w326) -> (w323:i32[])
            n205 = property on="Listbox" class="LstBox (strict)"("Item Symbols"=w323) -> ()  [unwired: 2 in, 2 out]
          }
          frame True {
            w327 = 0 ("Top Row")
            n206 = property on="Listbox" class="LstBox (strict)"() -> ("Number of Rows"=w329:u32)  [unwired: 2 in, 2 out]
            n207 = Initialize Array(0, w329) -> (w328:i32[])
            n208 = property on="Listbox" class="LstBox (strict)"("Top Row"=w327, "Value"=w327, "Item Symbols"=w328) -> ()  [unwired: 2 in, 2 out]
          }
        }
      }
      event "Listbox": Key Down {
        n209 = event-data() -> ("VKey"=w333:T25)  [unwired: 1 in]
        n210 = case shown="\"Left\", \"Right\"" w333 {
          selector: w333 -> [w338 _]
          tunnel: eventvkey."Left" ("VKey") -> [w336 _]
          frame "Left", "Right" {
            n211 = Equal?(x=w336, y=w338) -> (x = y?=w337:bool)
            n212 = Select(t=0, s=w337, f=1) -> (s? t:f=w339:i32)
            n213 = property on="Listbox" class="LstBox (strict)"() -> ("Item Symbols"=w342:i32[])  [unwired: 2 in, 2 out]
            n214 = Replace Array Subset(array=w342, new element=w339, index="Listbox") -> (w341:i32[])
            n215 = property on="Listbox" class="LstBox (strict)"("Item Symbols"=w341) -> ()  [unwired: 2 in, 2 out]
          }
          frame Default {
          }
        }
      }
      event "DB Camera Config": Value Change {
        n216 = event-data() -> ("NewVal"=w346:bool)  [unwired: 1 in]
        n217 = case shown="False" w346 {
          tunnel: w345 -> [w355 _]
          tunnel: [w348 w366] -> w344
          tunnel: w343 -> [w347 w366]
          frame False {
            w362 = "Camera"
            w365 = FALSE ("Visible")
            n218 = local read "Camera Settings"() -> (w354:T4)
            n219 = Index Array(array=w355) -> (element=w358:cluster{string[]})  [unwired: 1 in]
            n220 = Unbundle(w354) -> ("Frame Rate"=w353:i32, "Compression"=w352:i32, "Size"=w356:u16)
            n221 = Unbundle(w358) -> (w357:string[])
            n222 = Index Array(array=w357, index=w356) -> (element=w351:string)
            n223 = call-poly <vilib>:"Write Key.vi"("section"=w362, "value"=w351, "key"="Size", "refnum"=w347) -> ("refnum out"=w364:T24)  [unwired: 2 in, 5 out]
            n224 = call-poly <vilib>:"Write Key.vi"("section"=w362, "value"=w353, "key"="FrameRate", "refnum"=w364) -> ("refnum out"=w363:T24)  [unwired: 1 in, 6 out]
            n225 = property on="Camera Settings" class="Clust (strict)"("Visible"=w365) -> ()  [unwired: 2 in, 2 out]
            n226 = local write "DB Camera Config"(w365) -> ()
            n227 = call-poly <vilib>:"Write Key.vi"("section"=w362, "value"=w352, "key"="Compression", "refnum"=w363) -> ("refnum out"=w349:T24)  [unwired: 1 in, 6 out]
            n228 = call <vilib>:"Close Config Data.vi"("refnum"=w349) -> ("file path"=w350:path)  [unwired: 2 in, 8 out]
            n229 = call <vilib>:"Open Config Data.vi"("configuration file path"=w350) -> ("refnum"=w348:T24)  [unwired: 8 in, 2 out]
          }
          frame True {
            n230 = property on="Camera Settings" class="Clust (strict)"("Visible"=TRUE) -> ()  [unwired: 2 in, 2 out]
          }
        }
      }
      event "Camera Settings": Value Change {
        n231 = event-data() -> ("NewVal"=w379:T4)  [unwired: 1 in]
        n232 = Index Array(array=w375) -> (element=w374:cluster{string[]})  [unwired: 1 in]
        n233 = Unbundle(w379) -> ("Frame Rate"=w370:i32, "Compression"=w369:i32, "Size"=w372:u16)
        n234 = Unbundle(w374) -> (w373:string[])
        n235 = Index Array(array=w373, index=w372) -> (element=w371:string)
        n236 = Format Into String(format string="%s   %dfps   %d%%", w371, w370, w369) -> (resulting string=w376:string)  [unwired: 2 in, 1 out]
        n237 = Build Array(w376) -> (w377:string[])
        n238 = property on="DB Camera Config" class="Bool (strict)"("Strings [4]"=w377) -> ()  [unwired: 2 in, 2 out]
      }
      event "Motor.Enable": Value Change {
        n239 = event-data() -> ("NewVal"=w385:bool)  [unwired: 1 in]
        n240 = Unbundle("Motor") -> ("Value"=w384:dbl)  [unwired: 1 out]
        n241 = Select(t=w384, s=w385, f=0.0) -> (s? t:f=w382:dbl)
        n242 = call <vilib>:"NT Write Number.vi"("Numeric"=w382, "Name"=w381) -> ()  [unwired: 9 in, 1 out]
      }
      event "Test Slider": Value Change {
        n243 = event-data() -> ("NewVal"=w388:dbl)  [unwired: 1 in]
        n244 = call <vilib>:"NT Write Number.vi"("Numeric"=w388, "Name"=w389) -> ()  [unwired: 9 in, 1 out]
      }
      event "On/Off": Value Change {
        n245 = event-data() -> ("NewVal"=w393:bool)  [unwired: 1 in]
        n246 = Boolean To (0,1)(Boolean=w393) -> (0, 1=w392:i16)
        n247 = call <vilib>:"NT Write Number.vi"("Numeric"=w392, "Name"=w391) -> ()  [unwired: 9 in, 1 out]
      }
      event "Rev/Fwd": Value Change {
        n248 = event-data() -> ("NewVal.Forward"=w401:bool, "NewVal.Reverse"=w400:bool)  [unwired: 1 in]
        n249 = Boolean To (0,1)(Boolean=w401) -> (0, 1=w397:i16)
        n250 = Boolean To (0,1)(Boolean=w400) -> (0, 1=w399:i16)
        n251 = Negate(x=w399) -> (-x=w398:i16)
        n252 = Add(x=w397, y=w398) -> (x+y=w396:i16)
        n253 = call <vilib>:"NT Write Number.vi"("Numeric"=w396, "Name"=w395) -> ()  [unwired: 9 in, 1 out]
      }
      event "Test Ring": Value Change {
        n254 = event-data() -> ("NewVal"=w405:u16)  [unwired: 1 in]
        n255 = property on="Test Ring" class="Ring (strict)"() -> ("Strings []"=w406:string[])  [unwired: 2 in, 2 out]
        n256 = Index Array(array=w406, index=w405) -> (element=w404:string)
        n257 = call <vilib>:"NT Write String.vi"("String"=w404, "Name"=w403) -> ()  [unwired: 9 in, 1 out]
      }
      event "Rec Mode": Value Change {
        # "Update globals for recording mode and path to read log from.\nClear when logging and let NetworkTables set path for vision to\nuse."
        n258 = event-data() -> ("NewVal"=w416:enum32{"Stop", "Record", "Playback"})  [unwired: 1 in]
        n259 = global write "WPI_DashboardLogging Global.vi" "Logging Filename"(path "") -> ()
        n260 = case shown="\"Stop\", \"Record\"" w416 {
          tunnel: w415 -> [_ w418 w426]
          tunnel: [_ _ w425] -> w412
          tunnel: [_ _ w424] -> _
          tunnel: w410 -> [_ _ w422]
          tunnel: cluster{i32, i32} {-250, 170} -> [_ _ w421]
          tunnel: [_ _ T26 {"Image Size"=TRUE, "Image Type"=TRUE, "Pixel Value"=TRUE, "ROI Information"=TRUE, "Zoom Factor"=FALSE} ("Image Information Shown:All Elements")] -> w408
          tunnel: [_ _ TRUE ("Zoom Factor")] -> w407
          frame Default {
          }
          frame "Stop", "Record" {
            # "Place Window too"
            n261 = invoke class="VI" method="FP.Close"(reference=w418) -> (reference out=w417:refnum<vi>)  [unwired: 2 in, 2 out]
            n262 = invoke class="VI" method="Abort VI"(reference=w417) -> ()  [unwired: 2 in, 3 out]
          }
          frame "Playback" {
            n263 = call "Open Playback Panel.vi"("Offset"=w421, "DB VI Ref"=w422, "Playback in"=w426) -> ("Playback out"=w423:refnum<vi>)  [unwired: 8 in]
            n264 = register-events(w423) -> (reference out=w425:refnum<event-registration>, error out=w424:errorcluster)  [unwired: 2 in]
          }
        }
        n265 = global write "WPI_DashboardLogging Global.vi" "Recording"(w416) -> ()
        n266 = property on="Camera Image" class="ImageControl"("Image Information Shown"=w408, "Image Information Visible"=w407) -> ()  [unwired: 2 in, 2 out]
        n267 = call <vilib>:"WPI_DashboardNT Log FieldName Cache.vi"("Operation"=enum16{"Lookup/Add", "Index", "Clear"}."Clear") -> ()  [unwired: 8 in, 3 out]
      }
      event Panel Close {
        w427 = enum32{"Stop", "Record", "Playback"}."Stop" ("Rec Mode")
        n268 = event-data() -> ()  [unwired: 1 in, 4 out]
        n269 = local write "Rec Mode"(w427) -> ()
        n270 = global write "WPI_DashboardLogging Global.vi" "Recording"(w427) -> ()
      }
      event Panel Close {
        # "Abort playback window and ourself"
        n271 = event-data() -> ()  [unwired: 1 in, 4 out]
        n272 = invoke class="VI" method="FP.Close"(reference=w432) -> (reference out=w431:refnum<vi>)  [unwired: 2 in, 2 out]
        n273 = invoke class="VI" method="Abort VI"(reference=w431) -> (error out=w430:errorcluster)  [unwired: 2 in, 2 out]
        n274 = invoke class="VI" method="Abort VI"(error in=w430) -> ()  [unwired: 2 in, 3 out]
      }
    }
  }
  n275 = property on="On/Off" class="Bool (strict)"("Visible"=w25) -> ()  [unwired: 2 in, 2 out]
  n276 = property on="Motor" class="Clust (strict)"("Visible"=w25) -> ()  [unwired: 2 in, 2 out]
  n277 = property on="Progress" class="Clust (strict)"("Visible"=w25) -> ()  [unwired: 2 in, 2 out]
  n278 = property on="Test Ring" class="Ring (strict)"("Visible"=w25) -> ()  [unwired: 2 in, 2 out]
  n279 = property on="Rev/Fwd" class="Clust (strict)"("Visible"=w25) -> ()  [unwired: 2 in, 2 out]
  n280 = property on="Camera Settings" class="Clust (strict)"("Visible"=w25) -> ()  [unwired: 2 in, 2 out]
  n281 = local write "DB Camera Config"(w25) -> ()
  n282 = global write "WPI_DashboardLogging Global.vi" "Recording"(w8) -> ()
  n283 = local write "Rec Mode"(w8) -> ()
